vi "AIT 1553 - Create RT FIFOs.vi"(6 "FIFO Idx Qs":T2, 8 "error in (no error)":errorcluster, 11 "input cluster":T1) -> (0 "error out":errorcluster, 3 "output cluster":T1)   [LabVIEW 2013, in "AIT 1553 Custom Device.lvlib"]
uses:
  AIT 1553 Custom Device.lvlib
  RT Controls/FIFO Idx Qs.ctl
  RT Controls/FIFO.ctl
  RT Controls/Data Ref FGV Command.ctl
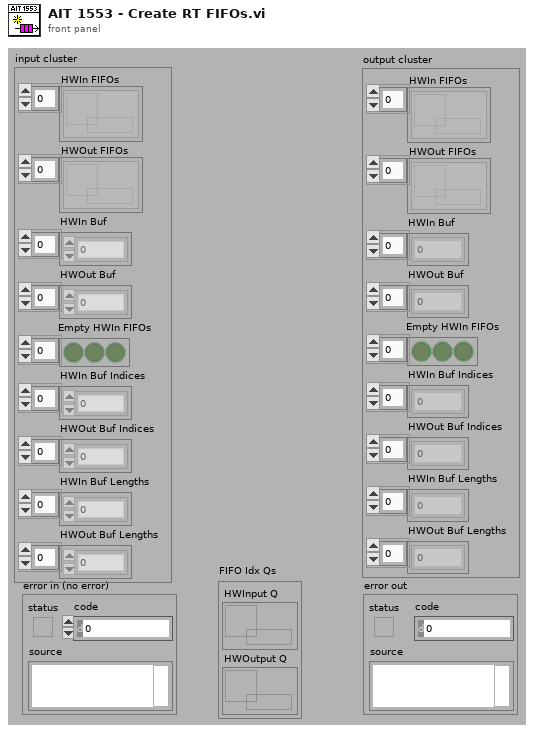
[diagram p1: front panel]
types:
  T1 = typedef "AIT 1553 Custom Device.lvlib/FIFO.ctl" = cluster{"HWIn FIFOs":refnum<k33>[], "HWOut FIFOs":refnum<k33>[], "HWIn Buf":dbl[], "HWOut Buf":dbl[], "Empty HWIn FIFOs":bool[], "HWIn Buf Indices":i32[], "HWOut Buf Indices":i32[], "HWIn Buf Lengths":i32[], "HWOut Buf Lengths":i32[]}
  T2 = typedef "AIT 1553 Custom Device.lvlib/FIFO Idx Qs.ctl" = cluster{"HWInput Q":refnum<queue>, "HWOutput Q":refnum<queue>}
  T3 = typedef "AIT 1553 Custom Device.lvlib/Data Ref FGV Command.ctl" = enum16{"Intialize", "Get", "Update"}
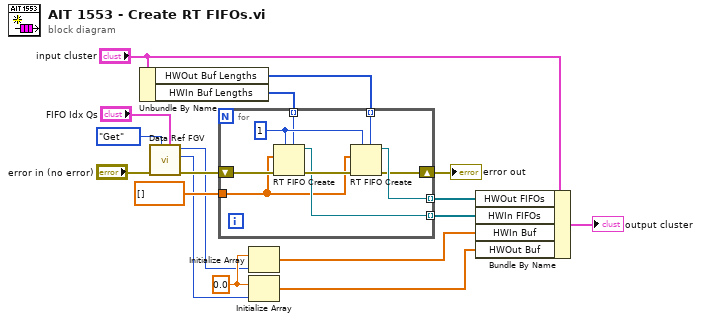
[diagram p0: block diagram]
diagram:
  w11 = 0.0
  n1 = Unbundle By Name("input cluster") -> ("HWOut Buf Lengths"=w6:i32[], "HWIn Buf Lengths"=w10:i32[])
  n2 = call "Data Ref FGV.vi"("FIFO Idx Qs"="FIFO Idx Qs", "Command"=Data_Ref_FGV_Command."Get", "error in (no error)"="error in (no error)") -> ("error out"=w16:errorcluster, "HWOutput FIFO Index / Length"=w3:i32, "HWInput FIFO Index / Length"=w4:i32)  [unwired: 6 in]
  n3 = for {
    tunnel: [w24] -> w9 mode=indexing
    tunnel: [w23] -> w2 mode=indexing
    tunnel: dbl[] [] -> [w21]
    tunnel: w10 -> [w19] mode=indexing
    tunnel: w6 -> [w18] mode=indexing
    shift-right: [w20] -> w1
    shift-left: w16 -> [w26]
    w22 = u32 1 ("size (10)")
    n4 = RT FIFO Create(1:w21, 3:w26, 4:w22, 6:w19) -> (8:w24:refnum<k33>, 11:w25:errorcluster)  [unwired: 4 in, 1 out]
    n5 = RT FIFO Create(1:w21, 3:w25, 4:w22, 6:w18) -> (8:w23:refnum<k33>, 11:w20:errorcluster)  [unwired: 4 in, 1 out]
  }
  "error out" <- w1
  n6 = Initialize Array(w11, w4) -> (w8:dbl[])
  n7 = Initialize Array(w11, w3) -> (w7:dbl[])
  n8 = Bundle By Name(cluster="input cluster", "HWOut FIFOs"=w2, "HWIn FIFOs"=w9, "HWIn Buf"=w8, "HWOut Buf"=w7) -> (→"output cluster":T1)
